vi "niRFUtil MT UTIL IQ Impairments Gain Imbalance.vi"(0 "Waveform In":T1={"x0"=0.0, "dx"=1.0, "y"=[]} caption="input complex waveform" {"y" format="%.2f"; "dx" format="%^.2e"; "x0" format="%^.2e"}, 2 "IQ Gain Imbalance, dB":dbl format="%.2f", 11 "error in (no error)":errorcluster) -> (4 "Waveform Out":T1 caption="output complex waveform" {"y" format="%.2f"; "dx" format="%^.2e"; "x0" format="%^.2e"}, 15 "error out":errorcluster)   [LabVIEW 2015, in "niRFUtil.lvlib"]
doc: "Performs the Gain Imbalance operation for IQ Impairment of an Input Data Waveform."
uses:
  niRFUtil.lvlib
  Includes/niRFUtil INC Complex Waveform.ctl
  Includes/niRFUtil INC Complex Array.ctl
  <vilib>/Analysis/5stat.llb/RMS (DBL).vi
  <vilib>/Analysis/NI_AALPro.lvlib
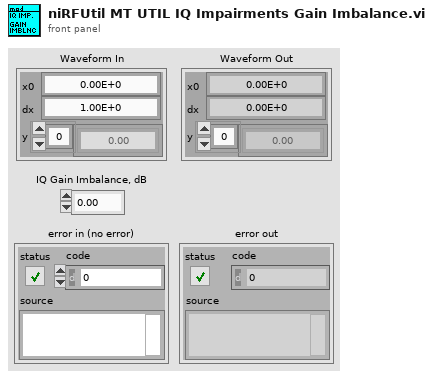
[diagram p1: front panel]
types:
  T1 = typedef "niRFUtil.lvlib/niRFUtil INC Complex Waveform.ctl" = cluster{"x0":dbl, "dx":dbl, "y":T2}
  T2 = typedef "niRFUtil.lvlib/niRFUtil INC Complex Array.ctl" = csg[]
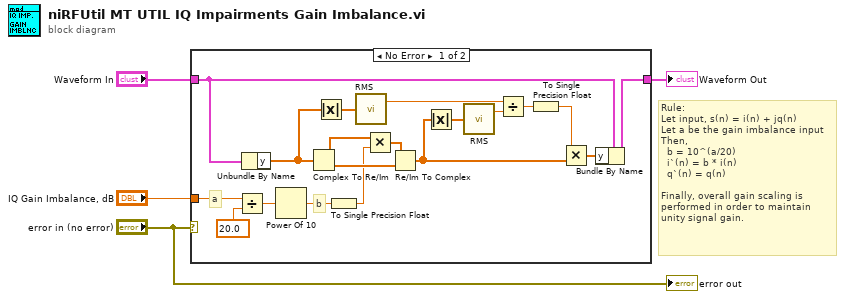
[diagram p0: block diagram]
diagram:
  # "Rule:\nLet input, s(n) = i(n) + jq(n)\nLet a be the gain imbalance input\nThen,\n  b = 10^(a/20)\n  i`(n) = b * i(n)\n  q`(n) = q(n)\n\nFinally, overall gain scaling is\nperformed in order to maintain\nunity signal gain."
  n1 = case shown="No Error" "error in (no error)" {
    tunnel: "IQ Gain Imbalance, dB" -> [w17 _]
    tunnel: "Waveform In" -> [w19 w24]
    tunnel: [w18 w24] -> w1
    frame No Error {
      # "a"
      # "b"
      n2 = Divide(x=w17, y=20.0) -> (x/y=w22:dbl)
      n3 = Unbundle By Name(w19) -> ("y"=w15:T2)
      n4 = Power Of 10(x=w22) -> (10^x=w8:dbl)
      n5 = Complex To Re/Im(x + iy=w15) -> (x=w21:sgl[], y=w7:sgl[])
      n6 = Absolute Value(x=w15) -> (abs(x)=w16:sgl[])
      n7 = To Single Precision Float(number=w8) -> (single precision float=w6:sgl)
      n8 = call-poly <vilib>:"RMS.vi"("X"=w16) -> ("rms value"=w11:dbl)  [unwired: 1 out]
      n9 = Multiply(x=w21, y=w6) -> (x*y=w20:sgl[])
      n10 = Re/Im To Complex(1:w7, 2:w20) -> (0:w13:csg[])
      n11 = Absolute Value(x=w13) -> (abs(x)=w14:sgl[])
      n12 = call-poly <vilib>:"RMS.vi"("X"=w14) -> ("rms value"=w12:dbl)  [unwired: 1 out]
      n13 = Divide(x=w11, y=w12) -> (x/y=w9:dbl)
      n14 = To Single Precision Float(number=w9) -> (single precision float=w5:sgl)
      n15 = Multiply(x=w5, y=w13) -> (x*y=w10:csg[])
      n16 = Bundle By Name(cluster=w19, "y"=w10) -> (w18:T1)
    }
    frame Error {
    }
  }
  "Waveform Out" <- w1
  "error out" <- "error in (no error)"
